vi "Connection Handler Worker.vi"(9 "Additional Data":variant, 10 "connection ID":T1, 11 "TCP Server Refnum":refnum<class "JKI TCP Server.lvclass">) -> ()   [LabVIEW 2020, in "CSM-TCP-Router.lvlib"]
uses:
  CSM-TCP-Router.lvlib
  <vilib>/addons/_JKI.lib/_JKI_lib_TCP_Server.llb/TCP Server Connection Session ID Cluster.ctl
  <vilib>/addons/_JKI.lib/_JKI_lib_TCP_Server.llb/JKI TCP Server.lvclass
  tcp-msg type.ctl
  20ff867f-262a-4864-b042-c50abd455195.vi
  9f8653f6-ccbf-4dca-88e7-a4c531b7661f.vi
  bd168d05-2ccd-4f69-90c9-be1b4e621865.vi
  316abe05-dd11-44a4-98b3-32ea1594dc48.vi
  a7f8194b-54d4-448d-8a65-d0b66a8fd47c.vi
  8a9da1d4-9237-4126-a3a1-8a9d876b672d.vi
  66683ee4-8938-4a2b-95b9-1d8ed72716c9.vi
  <userlib>/_NEVSTOP/Communicable State Machine(CSM)/AdvanceAPI/CSM - Revert Arguments-Safe String.vi
  <userlib>/_NEVSTOP/Communicable State Machine(CSM)/AdvanceAPI/CSM - Make String Arguments Safe.vi
  <userlib>/_NEVSTOP/Communicable State Machine(CSM)/AdvanceAPI/CSM - Compact Multiple States.vi
  <userlib>/_NEVSTOP/Communicable State Machine(CSM)/AdvanceAPI/CSM - Keywords.vi
  <userlib>/_NEVSTOP/Communicable State Machine(CSM)/addons/API-String-Arugments-Support/_Support/Data To API String Arguments.vi
  <userlib>/_NEVSTOP/Communicable State Machine(CSM)/_Shared/Trim Single-line Text.vi
  <userlib>/_NEVSTOP/Communicable State Machine(CSM)/addons/API-String-Arugments-Support/_Support/Query Data as API String Arguments(variant).vi
  <userlib>/_NEVSTOP/Communicable State Machine(CSM)/addons/API-String-Arugments-Support/_Support/Convert API String Arguments to Data(variant).vi
  <userlib>/_NEVSTOP/Communicable State Machine(CSM)/Communicable State Machine.lvlib
  <userlib>/_NEVSTOP/Communicable State Machine(CSM)/_csmHelper/API with lvcsm Support/CSM-Helper API with lvcsm Support.lvlib
  <userlib>/_NEVSTOP/Communicable State Machine(CSM)/_Shared/CSM Shared.lvlib
  <userlib>/_NEVSTOP/Communicable State Machine(CSM)/AdvanceAPI/CSM - Broadcast Message Type.ctl
panel:
  out "State History":string
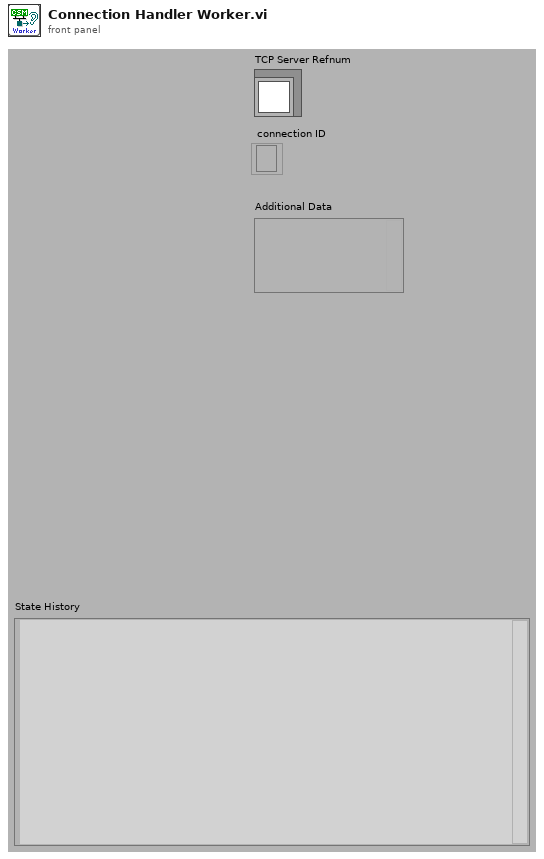
[diagram p1: front panel]
types:
  T1 = typedef "JKI TCP Server.lvclass/TCP Server Connection Session ID Cluster.ctl" = refnum<k5>
  T2 = typedef "CSM-TCP-Router.lvlib/tcp-msg type.ctl" = enum8{"info", "error", "cmd", "cmd-resp", "resp", "async-resp", "status", "interrupt"}
  T3 = typedef "Communicable State Machine.lvlib/CSM - Broadcast Message Type.ctl" = enum16{"<Null>", "Status", "Interrupt"}
  T4 = enum32{"Invalid", "Standard", "Closed", "Hidden", "Minimized", "Maximized"}
  T5 = enum32{"invalid app kind", "Development System", "Run Time System", "Student Edition", "Embedded LabVIEW", "Evaluation", "Custom"}
  T6 = typedef "Communicable State Machine.lvlib/_CSM_Response Source Message.ctl" = cluster{"‘State":string, "’Arguments":string, "’Error":errorcluster}
  T7 = cluster{"Current VI Reference":refnum<vi>, "Close Panel on Exit?":bool}
  T8 = cluster{"Core":cluster{"Current VI Reference":refnum<vi>, "Close Panel on Exit?":bool}, "Your Boolean data":bool}
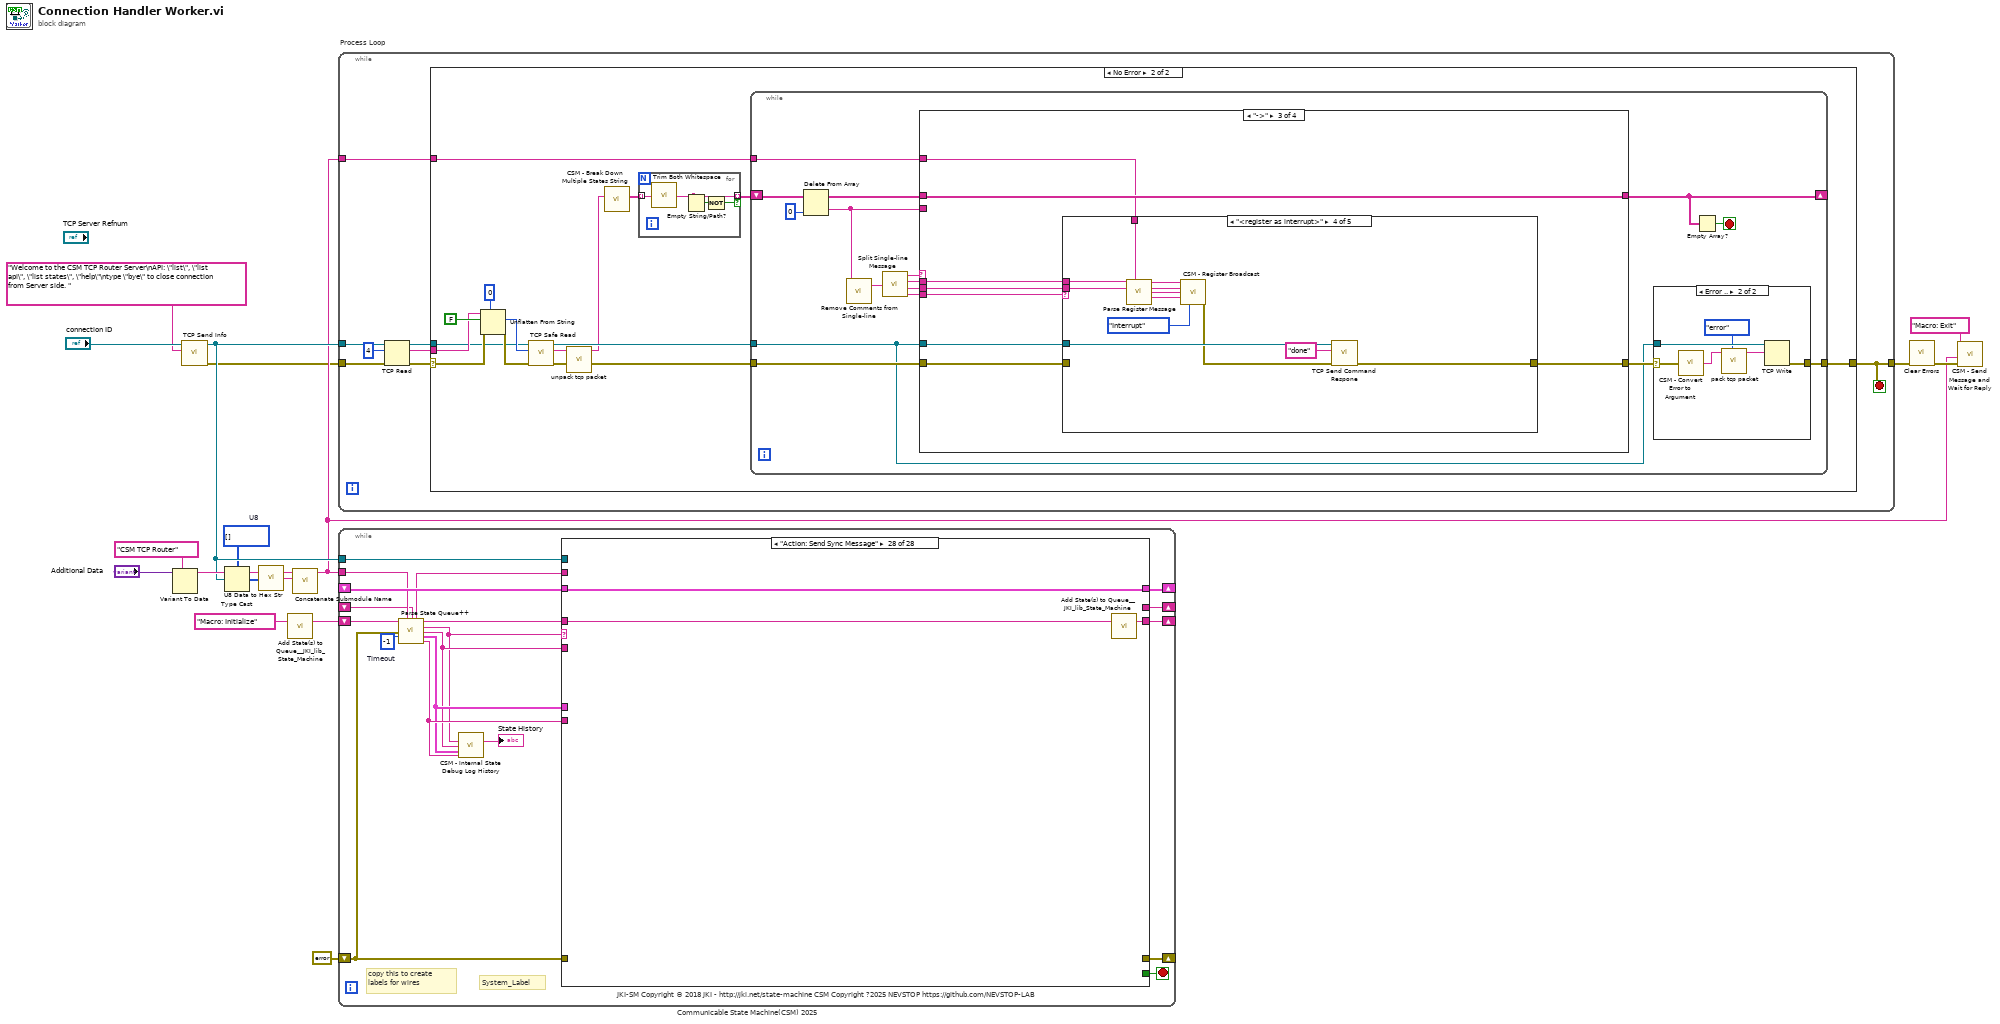
[diagram p0: block diagram]
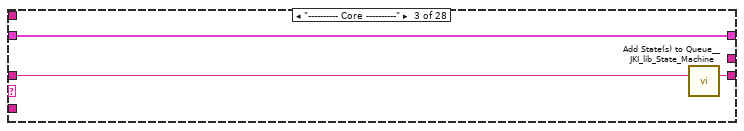
[diagram p4: hidden frame]
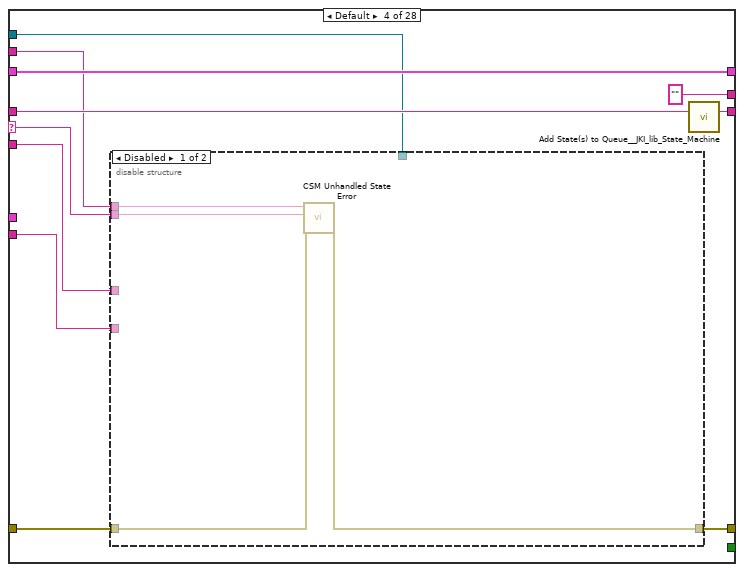
[diagram p5: hidden frame]
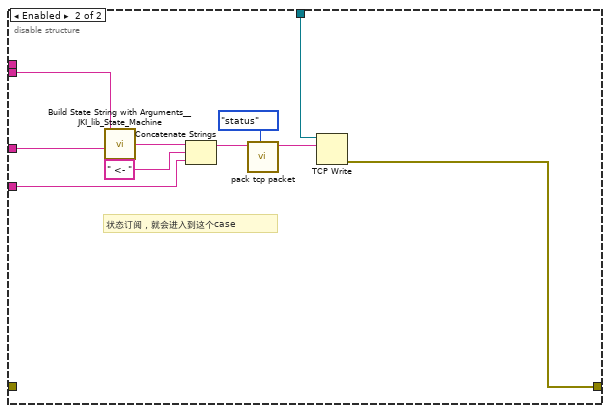
[diagram p6: hidden frame]
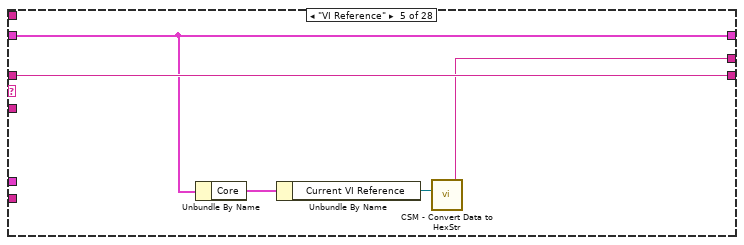
[diagram p7: hidden frame]
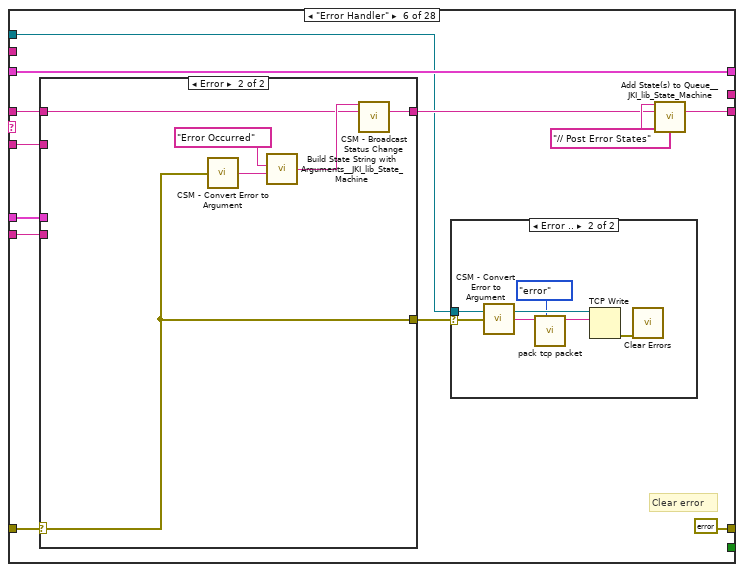
[diagram p8: hidden frame]
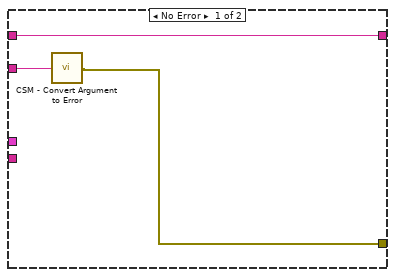
[diagram p10: hidden frame]
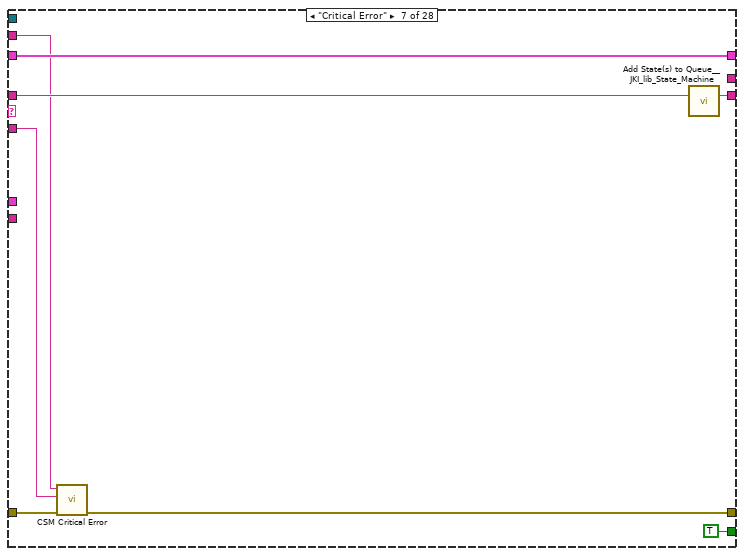
[diagram p11: hidden frame]
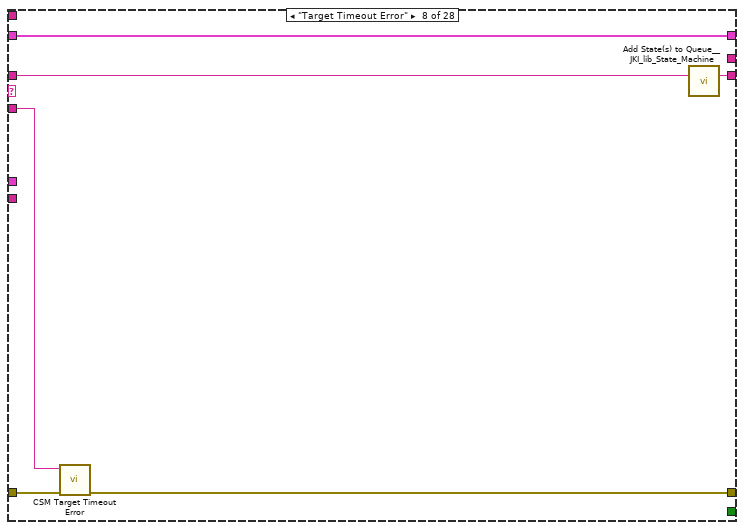
[diagram p12: hidden frame]
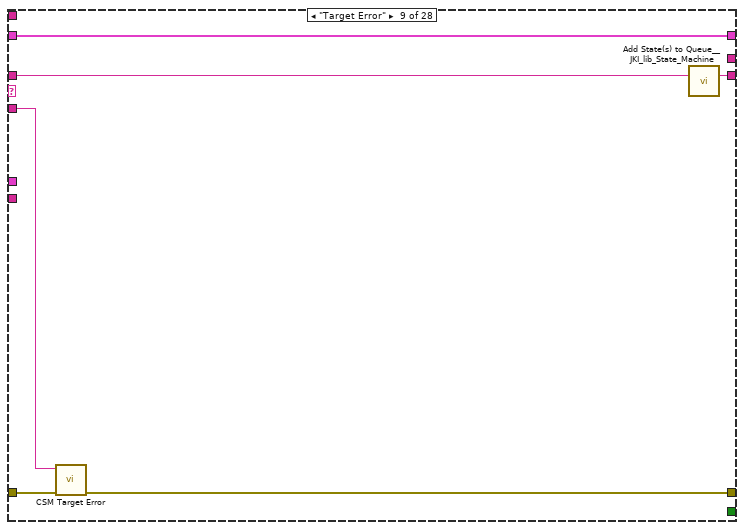
[diagram p13: hidden frame]
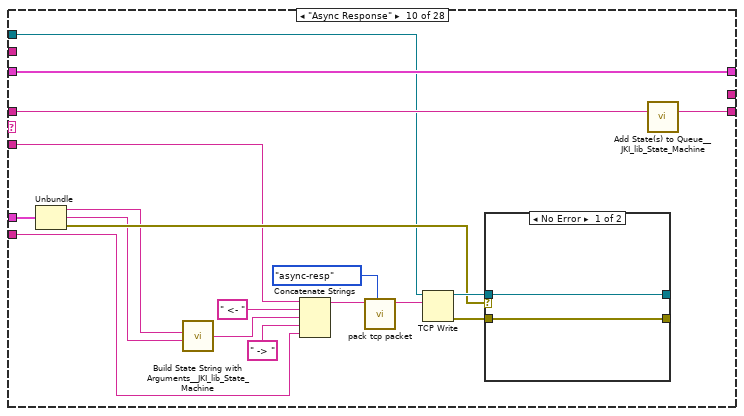
[diagram p14: hidden frame]
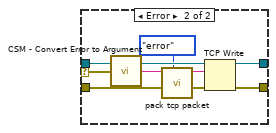
[diagram p15: hidden frame]
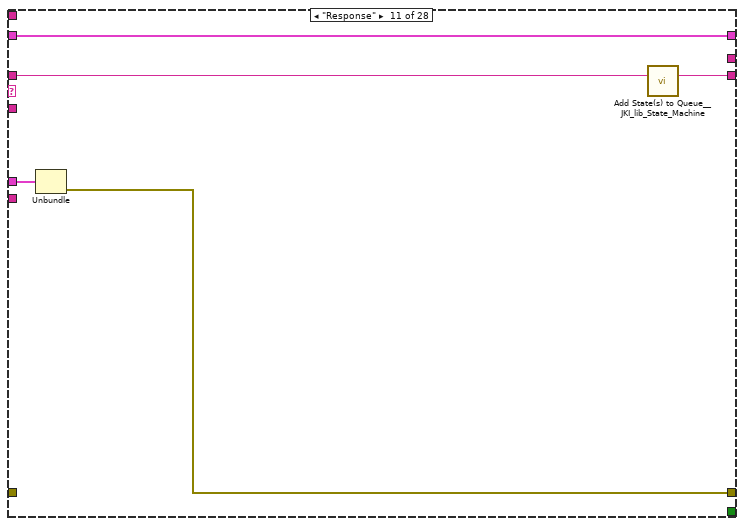
[diagram p16: hidden frame]
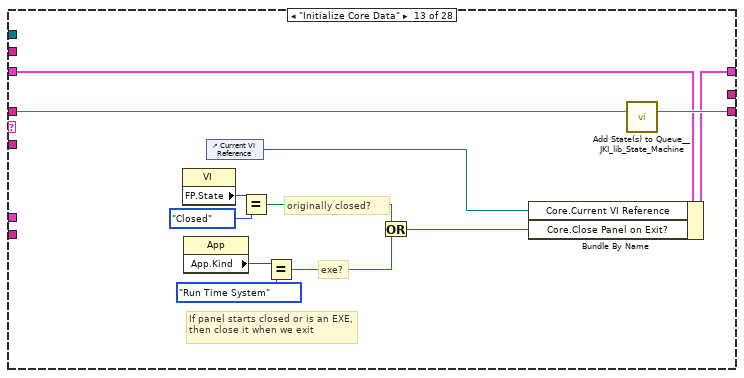
[diagram p18: hidden frame]
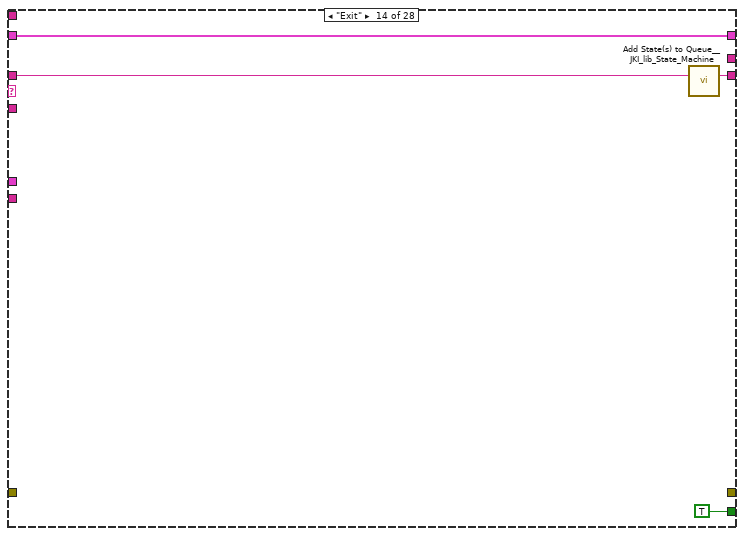
[diagram p19: hidden frame]
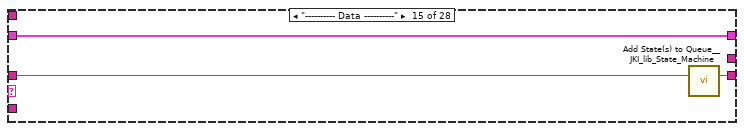
[diagram p20: hidden frame]
diagram:
  w5 = u8[] []  # U8
  n1 = Variant To Data(type="CSM TCP Router" ("Name(\"\" to use uuid)"), Variant="Additional Data") -> (data=w9:string)  [unwired: 1 in, 1 out]
  n2 = call "TCP Send Info.vi"("data in"="Welcome to the CSM TCP Router Server\nAPI: \"list\", \"list api\", \"list states\", \"help\"\ntype \"bye\" to close connection from Server side. ", "TCP Network Connection in"="connection ID") -> ("error out"=w2:errorcluster, "TCP Network Connection out"=w7:T1)  [unwired: 8 in]
  n3 = Type Cast(type=w5, x=w7) -> (*(type *) &x=w4:u8[])
  n4 = call <userlib>:"U8 Data to Hex Str.vi"("U8 Data[]"=w4) -> ("HEX String (0-9,A-F)"=w6:string)
  n5 = call <vilib>:"Add State(s) to Queue__JKI_lib_State_Machine.vi"("State(s) in (\"\")"="Macro: Initialize" ("Init States(\"Macro: Initialize\")")) -> ("States Out"=w15:string)  [unwired: 14 in]
  n6 = call <userlib>:"Concatenate Submodule Name.vi"("Module Name"=w6, "Group Name"=w9) -> ("Submodule Name"=w3:string)  [unwired: 9 in]
  n7 = while "Process Loop" {
    tunnel: w7 -> [w25]
    tunnel: [w21] -> w13
    tunnel: w3 -> [w20]
    tunnel: w2 -> [w18]
    stop <- w21 stop-if-true
    n8 = TCP Read(connection ID=w25, bytes to read=4, error in (no error)=w18) -> (connection ID out=w24:T1, data out=w22:string, error out=w23:errorcluster)  [unwired: 2 in]
    n9 = case shown="No Error" w23 {
      selector: w23 -> [w27 w37]
      tunnel: w24 -> [_ w30]
      tunnel: w22 -> [_ w38]
      tunnel: [w26 w44] -> w21
      tunnel: w20 -> [_ w41]
      frame Error {
        n10 = Unbundle By Name(w27) -> ("code"=w28:i32)
        n11 = case shown="56" w28 {
          tunnel: w27 -> [w29 _]
          tunnel: [w29 _] -> w26
          frame 0, Default {
          }
          frame 56 {
          }
        }
      }
      frame No Error {
        n12 = Unflatten From String(type=0, binary string=w38, data includes array or string size? (T)=FALSE, error in (no error)=w37) -> (value=w33:i32, error out=w36:errorcluster)  [unwired: 2 out]
        n13 = call "TCP Safe Read.vi"("error in (no error)"=w36, "bytes to read"=w33, "TCP Network Connection in"=w30) -> ("error out"=w35:errorcluster, "String"=w32:string, "TCP Network Connection out"=w34:refnum<k5>)  [unwired: 6 in]
        n14 = call "unpack tcp packet.vi"("TCP Pack"=w32) -> ("String"=w31:string)  [unwired: 9 in, 1 out]
        n15 = call <userlib>:"CSM - Break Down Multiple States String.vi"("States"=w31) -> ("Multiple States"=w43:string[])  [unwired: 10 in]
        n16 = for {
          tunnel: w43 -> [w48] mode=indexing
          tunnel: [w47] -> w42 mode=indexing if=w45
          n17 = call <userlib>:"Trim Both Whitespace.vi"("String"=w48) -> ("Trimmed String"=w47:string)  [unwired: 1 in]
          n18 = Empty String/Path?(string/path=w47) -> (empty?=w46:bool)
          n19 = Not(x=w46) -> (.not. x?=w45:bool)
        }
        n20 = while {
          tunnel: w34 -> [w51]
          tunnel: w35 -> [w64]
          tunnel: [w52] -> w44
          shift-right: [w54] -> _
          shift-left: w42 -> [w58]
          tunnel: w41 -> [w49]
          stop <- w55 stop-if-true
          n21 = Delete From Array(array=w58, index=0) -> (deleted portion=w50:string, array with subset deleted=w57:string[])  [unwired: 1 in]
          n22 = call <userlib>:"Remove Comments from Single-line.vi"("single-line text"=w50) -> ("single-line text without comments"=w63:string)  [unwired: 2 in]
          n23 = call <userlib>:"Split Single-line Message.vi"("single-line text"=w63) -> ("operator"=w62:string, "state"=w61:string, "args"=w60:string, "source/target"=w59:string)  [unwired: 6 in]
          n24 = case shown="\"->\"" w62 {
            selector: w62 -> [w75 _ _ _]
            tunnel: w51 -> [w81 w192 w196 w263]
            tunnel: [w80 w191 w200 w267] -> w53
            tunnel: w64 -> [w79 w184 w198 w265]
            tunnel: w61 -> [w78 w186 w195 w262]
            tunnel: w60 -> [w77 w185 w194 w261]
            tunnel: w59 -> [w76 w187 w193 w260]
            tunnel: [w74 w189 w199 w266] -> w54
            tunnel: w57 -> [w73 w189 w199 w266]
            tunnel: w50 -> [_ _ _ _]
            tunnel: w49 -> [w72 w188 w197 w264]
            frame Default {
              n25 = case shown="Default" w78 {
                selector: w78 -> [w89 _ _ _ _ _ _ _]
                tunnel: w81 -> [w92 w97 w107 w120 w133 w146 w160 w180]
                tunnel: [w91 errorcluster {"status"=TRUE, "code"=0, "source"=""} ("error out") w102 w119 w132 w145 w162 w181] -> w80
                tunnel: w79 -> [w84 w98 w106 _ _ _ w161 w178]
                tunnel: w77 -> [w90 _ _ w115 w128 w141 _ _]
                tunnel: w76 -> [_ _ _ _ _ _ _ _]
                tunnel: w75 -> [_ _ _ _ _ _ _ _]
                tunnel: [w88 w95 w101 w118 w131 w144 w168 w182] -> w74
                tunnel: w73 -> [w88 w95 w101 w118 w131 w144 w168 w182]
                tunnel: w72 -> [_ _ _ w114 w127 w140 w163 _]
                frame Default {
                  n26 = call <vilib>:"Build State String with Arguments__JKI_lib_State_Machine.vi"("Arguments (\"\")"=w90, "State"=w89) -> ("State with Arguments"=w85:string)  [unwired: 4 in]
                  n27 = Format Into String(format string="You typed \"%s\", which is not recognized as a command", w85) -> (resulting string=w86:string)  [unwired: 2 in, 1 out]
                  n28 = call "pack tcp packet.vi"("tcp-message-type"=tcp-msg_type."error", "String"=w86) -> ("TCP Pack"=w83:string)  [unwired: 9 in]
                  n29 = TCP Write(connection ID=w92, data in=w83, error in (no error)=w84) -> (error out=w91:errorcluster)  [unwired: 1 in, 2 out]
                }
                frame "bye", "exit", "quit" {
                  n30 = call "TCP Send Info.vi"("error in (no error)"=w98, "data in"="Good bye.\r\n", "TCP Network Connection in"=w97) -> ("error out"=w94:errorcluster, "TCP Network Connection out"=w93:T1)  [unwired: 7 in]
                  n31 = TCP Close Connection(connection ID=w93, error in (no error)=w94) -> ()  [unwired: 1 in, 2 out]
                }
                frame "list", "list CSM", "List CSMs" {
                  n32 = call <userlib>:"CSM - List Modules.vi"("Error In"=w106) -> ("error out"=w104:errorcluster, "Module Names"=w105:string[])  [unwired: 9 in]
                  n33 = call "Convert Data To API String Arguments.vim"("error in (no error)"=w104, "Data"=w105) -> ("error out"=w103:errorcluster, "API String"=w100:string)  [unwired: 6 in]
                  n34 = call "TCP Send Response.vi"("error in (no error)"=w103, "Response"=w100, "connection ID"=w107) -> ("error out"=w102:errorcluster)  [unwired: 7 in, 1 out]
                }
                frame "list API", "list interface" {
                  n35 = call <userlib>:"CSM - Check If Module Exists.vi"("CSM Name"=w115) -> ("error out"=w117:errorcluster, "Exist?"=w112:bool, "CSM Name (Dup)"=w116:string)  [unwired: 8 in]
                  n36 = call "Error If Module Not Exist.vi"("Error in"=w117, "Module Exist?"=w112) -> ("Error out"=w113:errorcluster)  [unwired: 9 in]
                  n37 = call <userlib>:"Read CSM API with lvcsm Support.vi"("Current Module (\"\" to Generate an ID)"=w114, "error in (no error)"=w113, "CSM Name"=w116) -> ("error out"=w110:errorcluster, "CSMAPI List"=w109:string[])  [unwired: 7 in]
                  n38 = call "Convert Data To API String Arguments.vim"("error in (no error)"=w110, "Data"=w109) -> ("error out"=w111:errorcluster, "API String"=w108:string)  [unwired: 6 in]
                  n39 = call "TCP Send Response.vi"("error in (no error)"=w111, "Response"=w108, "connection ID"=w120) -> ("error out"=w119:errorcluster)  [unwired: 7 in, 1 out]
                }
                frame "List State", "List States" {
                  n40 = call <userlib>:"CSM - Check If Module Exists.vi"("CSM Name"=w128) -> ("error out"=w130:errorcluster, "Exist?"=w125:bool, "CSM Name (Dup)"=w129:string)  [unwired: 8 in]
                  n41 = call "Error If Module Not Exist.vi"("Error in"=w130, "Module Exist?"=w125) -> ("Error out"=w126:errorcluster)  [unwired: 9 in]
                  n42 = call <userlib>:"Read CSM States with lvcsm Support.vi"("Current Module (\"\" to Generate an ID)"=w127, "error in (no error)"=w126, "CSM Name"=w129) -> ("error out"=w121:errorcluster, "CSMAPI List"=w122:string[])  [unwired: 7 in]
                  n43 = call "Convert Data To API String Arguments.vim"("error in (no error)"=w121, "Data"=w122) -> ("error out"=w124:errorcluster, "API String"=w123:string)  [unwired: 6 in]
                  n44 = call "TCP Send Response.vi"("error in (no error)"=w124, "Response"=w123, "connection ID"=w133) -> ("error out"=w132:errorcluster)  [unwired: 7 in, 1 out]
                }
                frame "help" {
                  n45 = call <userlib>:"CSM - Check If Module Exists.vi"("CSM Name"=w141) -> ("error out"=w143:errorcluster, "Exist?"=w138:bool, "CSM Name (Dup)"=w142:string)  [unwired: 8 in]
                  n46 = call "Error If Module Not Exist.vi"("Error in"=w143, "Module Exist?"=w138) -> ("Error out"=w139:errorcluster)  [unwired: 9 in]
                  n47 = disable-structure shown="Enabled" {
                    disable-tunnel: w139 -> [w153 w158]
                    disable-tunnel: w142 -> [w152 w157]
                    disable-tunnel: [w150 w155] -> w135
                    disable-tunnel: [w148 w154] -> w134
                    disable-tunnel: w140 -> [w147 w156]
                    frame Disabled {
                      n48 = call <userlib>:"CSM - Module VI Reference.vi"("Current Module (\"\" to Generate an ID)"=w147, "error in (no error)"=w153, "CSM Name"=w152) -> ("error out"=w151:errorcluster, "CSM Module VIRef"=w149:refnum<vi>)  [unwired: 7 in]
                      n49 = property class="VI"(reference=w149, error in=w151) -> (error out=w150:errorcluster, "Description"=w148:string)  [unwired: 1 out]
                    }
                    frame Enabled {
                      n50 = call "Read CSM Doc.vi"("Current Module(\"\" to generate a ID)"=w156, "error in (no error)"=w158, "CSM Name"=w157) -> ("Error out"=w155:errorcluster, "CSM Doc"=w154:string)  [unwired: 7 in]
                    }
                  }
                  n51 = call "Convert Data To API String Arguments.vim"("error in (no error)"=w135, "Data"=w134) -> ("error out"=w137:errorcluster, "API String"=w136:string)  [unwired: 6 in]
                  n52 = call "TCP Send Response.vi"("error in (no error)"=w137, "Response"=w136, "connection ID"=w146) -> ("error out"=w145:errorcluster)  [unwired: 7 in, 1 out]
                }
                frame "Refresh lvcsm" {
                  n53 = call <userlib>:"CSM - List Modules.vi"("Error In"=w161) -> ("error out"=w167:errorcluster, "Module Names"=w166:string[])  [unwired: 9 in]
                  n54 = for {
                    tunnel: w167 -> [w177]
                    tunnel: w166 -> [w170] mode=indexing
                    tunnel: [w172] -> w165 mode=indexing
                    tunnel: w163 -> [w171]
                    n55 = call <userlib>:"Read CSM States with lvcsm Support.vi"("Current Module (\"\" to Generate an ID)"=w171, "error in (no error)"=w177, "Force? (F)"=TRUE ("Force?(F)"), "CSM Name"=w170) -> ("error out"=w176:errorcluster)  [unwired: 6 in, 1 out]
                    n56 = call <userlib>:"Read CSM API with lvcsm Support.vi"("Current Module (\"\" to Generate an ID)"=w171, "error in (no error)"=w176, "Force? (F)"=TRUE ("Force?(F)"), "CSM Name"=w170) -> ("error out"=w173:errorcluster)  [unwired: 6 in, 1 out]
                    n57 = call "Read CSM Doc.vi"("Current Module(\"\" to generate a ID)"=w171, "error in (no error)"=w173, "Force?(F)"=TRUE, "CSM Name"=w170) -> ("Error out"=w172:errorcluster)  [unwired: 6 in, 1 out]
                  }
                  n58 = Merge Errors(w165) -> (w164:errorcluster)
                  n59 = call "TCP Send Response.vi"("error in (no error)"=w164, "Response"="", "connection ID"=w160) -> ("error out"=w162:errorcluster)  [unwired: 7 in, 1 out]
                }
                frame "ping" {
                  n60 = call "TCP Send Response.vi"("error in (no error)"=w178, "Response"="pong", "connection ID"=w180) -> ("error out"=w181:errorcluster)  [unwired: 7 in, 1 out]
                }
              }
            }
            frame "-@" {
              n61 = call <userlib>:"CSM - Send Message and Wait for Reply.vi"("Current Module (\"\" to Generate an ID)"=w188, "Error In (No Error)"=w184, "Target Module"=w187, "Arguments (\"\")"=w185, "State"=w186) -> ("error out"=w183:errorcluster, "Response"=w190:string)  [unwired: 4 in, 1 out]
              n62 = call "TCP Send Response.vi"("error in (no error)"=w183, "Response"=w190, "connection ID"=w192) -> ("error out"=w191:errorcluster)  [unwired: 7 in, 1 out]
            }
            frame "->" {
              n63 = case shown="\"<register as interrupt>\"" w193 {
                selector: w193 -> [_ _ _ _ w250]
                tunnel: [w201 w213 w225 w237 w256] -> w200
                tunnel: w198 -> [_ _ _ _ w255]
                tunnel: w197 -> [w209 w220 w232 w244 w254]
                tunnel: w196 -> [w203 w215 w227 w239 w253]
                tunnel: w195 -> [w210 w221 w233 w245 w252]
                tunnel: w194 -> [w211 w222 w234 w246 w251]
                frame "<unregister>" {
                  n64 = call <userlib>:"Parse Unregister Message.vi"("State"=w210, "Module Name"=w209, "Args"=w211) -> ("Target"=w207:string, "Source"=w208:string, "Status"=w206:string, "Api"=w205:string)  [unwired: 8 in, 1 out]
                  n65 = call <userlib>:"CSM - Unregister Broadcast.vi"("CSM Name(Empty for Broadcast Event)"=w207, "Source CSM Name (* as Default)"=w208, "Trigger"=w206, "API (\"*\" as Default)"=w205) -> ("error out"=w202:errorcluster)  [unwired: 10 in, 1 out]
                  n66 = call "TCP Send Command Respone.vi"("error in (no error)"=w202, "Response"="done", "connection ID"=w203) -> ("error out"=w201:errorcluster)  [unwired: 7 in, 1 out]
                }
                frame "<register>" {
                  n67 = call <userlib>:"Parse Register Message.vi"("State"=w221, "Module Name"=w220, "Args"=w222) -> ("Target"=w218:string, "Source"=w219:string, "Status"=w217:string, "Api"=w216:string)  [unwired: 8 in, 1 out]
                  n68 = call <userlib>:"CSM - Register Broadcast.vi"("CSM Name(Empty for Broadcast Event)"=w218, "Source CSM Name (* as Default)"=w219, "Trigger"=w217, "API (If \"\", Same as Trigger)"=w216) -> ("error out"=w214:errorcluster)  [unwired: 10 in, 1 out]
                  n69 = call "TCP Send Command Respone.vi"("error in (no error)"=w214, "Response"="done", "connection ID"=w215) -> ("error out"=w213:errorcluster)  [unwired: 7 in, 1 out]
                }
                frame "<register as status>" {
                  n70 = call <userlib>:"Parse Register Message.vi"("State"=w233, "Module Name"=w232, "Args"=w234) -> ("Target"=w230:string, "Source"=w231:string, "Status"=w229:string, "Api"=w228:string)  [unwired: 8 in, 1 out]
                  n71 = call <userlib>:"CSM - Register Broadcast.vi"("CSM Name(Empty for Broadcast Event)"=w230, "Source CSM Name (* as Default)"=w231, "Trigger"=w229, "API (If \"\", Same as Trigger)"=w228, "Priority (No Change)"=CSM_-_Broadcast_Message_Type."Status") -> ("error out"=w226:errorcluster)  [unwired: 9 in, 1 out]
                  n72 = call "TCP Send Command Respone.vi"("error in (no error)"=w226, "Response"="done", "connection ID"=w227) -> ("error out"=w225:errorcluster)  [unwired: 7 in, 1 out]
                }
                frame "<register as interrupt>" {
                  n73 = call <userlib>:"Parse Register Message.vi"("State"=w245, "Module Name"=w244, "Args"=w246) -> ("Target"=w242:string, "Source"=w243:string, "Status"=w241:string, "Api"=w240:string)  [unwired: 8 in, 1 out]
                  n74 = call <userlib>:"CSM - Register Broadcast.vi"("CSM Name(Empty for Broadcast Event)"=w242, "Source CSM Name (* as Default)"=w243, "Trigger"=w241, "API (If \"\", Same as Trigger)"=w240, "Priority (No Change)"=CSM_-_Broadcast_Message_Type."Interrupt") -> ("error out"=w238:errorcluster)  [unwired: 9 in, 1 out]
                  n75 = call "TCP Send Command Respone.vi"("error in (no error)"=w238, "Response"="done", "connection ID"=w239) -> ("error out"=w237:errorcluster)  [unwired: 7 in, 1 out]
                }
                frame Default {
                  n76 = call <userlib>:"CSM - Request CSM to Post Message.vi"("Module Name"=w254, "Target Module (\"\" By Default)"=w250, "Arguments (\"\")"=w251, "State"=w252) -> ("error out"=w247:errorcluster)  [unwired: 7 in]
                  n77 = Merge Errors(w255, w247) -> (w248:errorcluster)
                  n78 = call "TCP Send Command Respone.vi"("error in (no error)"=w248, "Response"="Message posted", "connection ID"=w253) -> ("error out"=w256:errorcluster)  [unwired: 7 in, 1 out]
                }
              }
            }
            frame "->|" {
              n79 = call <userlib>:"CSM - Post Message.vi"("Current Module (\"\" to Generate an ID)"=w264, "Target Module"=w260, "Arguments (\"\")"=w261, "State"=w262) -> ("error out"=w258:errorcluster)  [unwired: 7 in]
              n80 = call "Synchronize Data Flow.vim"("input 2"=w265, "input 1"=w258) -> ("output 2"=w259:errorcluster)  [unwired: 2 in, 3 out]
              n81 = call "TCP Send Command Respone.vi"("error in (no error)"=w259, "Response"="No-Rep Message Posted", "connection ID"=w263) -> ("error out"=w267:errorcluster)  [unwired: 7 in, 1 out]
            }
          }
          n82 = case shown="Error .." w53 {
            selector: w53 -> [w65 w68]
            tunnel: w51 -> [_ w71]
            tunnel: [w65 w70] -> w52
            frame No Error {
            }
            frame Error {
              n83 = call <userlib>:"CSM - Convert Error to Argument.vi"("Error"=w68) -> ("Argument"=w69:string)  [unwired: 4 in]
              n84 = call "pack tcp packet.vi"("tcp-message-type"=tcp-msg_type."error", "String"=w69) -> ("TCP Pack"=w67:string)  [unwired: 9 in]
              n85 = TCP Write(connection ID=w71, data in=w67) -> (error out=w70:errorcluster)  [unwired: 2 in, 2 out]
            }
          }
          n86 = Empty Array?(array=w54) -> (empty?=w55:bool)
        }
      }
    }
  }
  n87 = while "Communicable State Machine(CSM) 2025" {
    shift-right: [w281] -> _
    shift-left: _ -> [w280]
    shift-right: [w284] -> _
    shift-left: errorcluster {"status"=FALSE, "code"=0, "source"=""} ("error out") -> [w270]
    shift-right: [w283] -> _
    shift-left: w15 -> [w285]
    tunnel: w3 -> [w277]
    shift-right: [w278] -> _
    shift-left: _ -> [w272]
    tunnel: w7 -> [w268]
    stop <- w282 stop-if-true
    w279 = -1  # Timeout
    # "copy this to create labels for wires"
    # "System_Label"
    # "JKI-SM Copyright © 2018 JKI - http://jki.net/state-machine CSM Copyright ?2025 NEVSTOP https://github.com/NEVSTOP-LAB"
    n88 = call <userlib>:"Parse State Queue++.vi"("State Queue"=w285, "Name (\"\" to Use UUID)"=w277, "Response Arguments"=w272, "Previous Error"=w270, "Dequeue (1 ms)"=w279) -> ("Name Used"=w271:string, "Remaining States"=w286:string, "Current State"=w273:string, "Arguments"=w274:string, "Additional Information"=w275:T6, "Source CSM"=w276:string)  [unwired: 5 in]
    n89 = call <userlib>:"CSM - Internal State Debug Log History.vi"("State"=w273, "Arguments (\"\")"=w274, ">> Response Source Message >>"=w275, "Source (\"\")"=w276) -> ("Debug Log"=→"State History":string)  [unwired: 11 in]
    n90 = case shown="\"Action: Send Sync Message\"" w273 {
      selector: w273 -> [_ _ _ w299 _ _ _ _ _ _ _ _ _ _ _ _ _ _ _ _ _ _ _ _ _ _ _ _]
      tunnel: w286 -> [w287 w290 w293 w302 w323 w329 w357 w363 w369 w386 w401 w405 w417 w421 w424 w429 w435 w440 w442 w447 w450 w454 w458 w460 w463 w467 w472 w475]
      tunnel: w274 -> [_ _ _ w295 _ w328 w351 w360 w366 w378 _ _ _ _ _ _ w430 w439 _ _ _ _ _ _ _ w465 _ _]
      tunnel: w280 -> [w288 w289 w291 w300 w320 w334 w355 w361 w367 w387 w402 w404 w411 w419 w422 _ w434 w438 w441 w443 w448 w452 w456 w459 w462 w466 w470 w473]
      tunnel: [_ _ _ w304 _ errorcluster {"status"=FALSE, "code"=0, "source"=""} ("error out") w358 w359 w365 _ w399 _ _ _ _ _ w431 w436 _ w444 _ _ _ _ _ _ _ _] -> w284
      tunnel: w270 -> [_ _ _ w303 _ w332 w353 w364 w370 _ _ _ _ _ _ _ _ _ _ _ _ _ _ _ _ _ _ _]
      tunnel: [w287 w290 w292 w301 w323 w330 w356 w362 w368 w388 w403 w405 w416 w420 w423 w428 w435 w440 w442 w446 w449 w453 w457 w460 w463 w467 w471 w474] -> w283
      tunnel: [_ _ _ _ _ _ TRUE _ _ _ _ _ _ TRUE _ _ _ _ _ _ _ _ _ _ _ _ _ _] -> w282
      tunnel: [w288 w289 w291 w300 w320 w334 w355 w361 w367 w387 w402 w404 w415 w419 w422 w427 w433 w437 w441 w443 w448 w452 w456 w459 w462 w466 w470 w473] -> w281
      tunnel: w276 -> [_ _ _ w294 _ w327 _ _ _ w371 _ _ _ _ _ _ _ _ _ _ _ _ _ _ _ _ _ _]
      tunnel: w275 -> [_ _ _ _ _ w326 _ _ _ w385 w400 _ _ _ _ _ _ _ _ _ _ _ _ _ _ _ _ _]
      tunnel: [_ _ _ "" w319 _ _ _ _ _ _ _ _ _ _ _ w432 _ _ _ _ _ _ _ "API1 Response" w464 _ _] -> w278
      tunnel: w271 -> [_ _ _ w297 _ _ w352 _ _ _ _ _ _ _ _ _ _ _ _ _ _ _ _ _ _ _ _ _]
      tunnel: w268 -> [_ _ _ w296 _ w324 _ _ _ w379 _ _ _ _ _ _ _ _ _ _ _ _ _ _ _ _ _ _]
      frame "", "Idle" {
      }
      frame "CSM Documentation" {
      }
      frame "---------- Core ----------" {
        n91 = call <vilib>:"Add State(s) to Queue__JKI_lib_State_Machine.vi"("State(s) in (\"\")"=w293) -> ("States Out"=w292:string)  [unwired: 14 in]
      }
      frame Default {
        n92 = disable-structure shown="Disabled" {
          disable-tunnel: [w308 w309] -> w304
          disable-tunnel: w303 -> [w307 _]
          disable-tunnel: w299 -> [w306 w313]
          disable-tunnel: w297 -> [w305 _]
          disable-tunnel: w296 -> [_ w314]
          disable-tunnel: w295 -> [_ w312]
          disable-tunnel: w294 -> [_ w310]
          frame Disabled {
            n93 = call <userlib>:"CSM Unhandled State Error.vi"("error in (no error)"=w307, "Undefined State"=w306, "CSM Name"=w305) -> ("error out"=w308:errorcluster)  [unwired: 8 in]
          }
          frame Enabled {
            # "状态订阅，就会进入到这个case"
            n94 = call <vilib>:"Build State String with Arguments__JKI_lib_State_Machine.vi"("Arguments (\"\")"=w312, "State"=w313) -> ("State with Arguments"=w311:string)  [unwired: 4 in]
            n95 = Concatenate Strings(w311, " <- " ("string"), w310) -> (w316:string)
            n96 = call "pack tcp packet.vi"("tcp-message-type"=tcp-msg_type."status", "String"=w316) -> ("TCP Pack"=w318:string)  [unwired: 9 in]
            n97 = TCP Write(connection ID=w314, data in=w318) -> (error out=w309:errorcluster)  [unwired: 2 in, 2 out]
          }
        }
        n98 = call <vilib>:"Add State(s) to Queue__JKI_lib_State_Machine.vi"("State(s) in (\"\")"=w302) -> ("States Out"=w301:string)  [unwired: 14 in]
      }
      frame "VI Reference" {
        n99 = Unbundle By Name(w320) -> ("Core"=w322:T7)
        n100 = Unbundle By Name(w322) -> ("Current VI Reference"=w321:refnum<vi>)
        n101 = call <userlib>:"CSM - Convert Data to HexStr.vi"("Variant"=w321) -> ("HEX String (0-9,A-F)"=w319:string)  [unwired: 8 in]
      }
      frame "Error Handler" {
        # "Clear error"
        n102 = case shown="Error" w332 {
          selector: w332 -> [_ w345]
          tunnel: [w344 w347] -> w331
          tunnel: w329 -> [w344 w346]
          tunnel: w328 -> [w343 _]
          tunnel: w327 -> [_ _]
          tunnel: w326 -> [_ _]
          tunnel: [w342 w345] -> w325
          frame No Error {
            n103 = call <userlib>:"CSM - Convert Argument to Error.vi"("Argument"=w343) -> ("Error"=w342:errorcluster)  [unwired: 4 in]
          }
          frame Error {
            n104 = call <userlib>:"CSM - Convert Error to Argument.vi"("Error"=w345) -> ("Argument"=w349:string)  [unwired: 4 in]
            n105 = call <vilib>:"Build State String with Arguments__JKI_lib_State_Machine.vi"("Arguments (\"\")"=w349, "State"="Error Occurred" ("Status with Arguments")) -> ("State with Arguments"=w348:string)  [unwired: 4 in]
            n106 = call <userlib>:"CSM - Broadcast Status Change.vi"("Status With Arguments"=w348, "State Queue"=w346) -> ("Remaining States"=w347:string)  [unwired: 13 in]
          }
        }
        n107 = case shown="Error .." w325 {
          selector: w325 -> [_ w339]
          tunnel: w324 -> [_ w341]
          frame No Error {
          }
          frame Error {
            n108 = call <userlib>:"CSM - Convert Error to Argument.vi"("Error"=w339) -> ("Argument"=w338:string)  [unwired: 4 in]
            n109 = call "pack tcp packet.vi"("tcp-message-type"=tcp-msg_type."error", "String"=w338) -> ("TCP Pack"=w337:string)  [unwired: 9 in]
            n110 = TCP Write(connection ID=w341, data in=w337) -> (error out=w340:errorcluster)  [unwired: 2 in, 2 out]
            n111 = call <vilib>:"Clear Errors.vi"("error in (no error)"=w340) -> ()  [unwired: 5 in, 2 out]
          }
        }
        n112 = call <vilib>:"Add State(s) to Queue__JKI_lib_State_Machine.vi"("State(s) in Front (\"\")"="// Post Error States", "State(s) in (\"\")"=w331) -> ("States Out"=w330:string)  [unwired: 13 in]
      }
      frame "Critical Error" {
        n113 = call <userlib>:"CSM Critical Error.vi"("error in (no error)"=w353, "Arugments (As Reason)"=w351, "CSM Name"=w352) -> ("error out"=w358:errorcluster)  [unwired: 8 in]
        n114 = call <vilib>:"Add State(s) to Queue__JKI_lib_State_Machine.vi"("State(s) in (\"\")"=w357) -> ("States Out"=w356:string)  [unwired: 14 in]
      }
      frame "Target Timeout Error" {
        n115 = call <userlib>:"CSM Target Timeout Error.vi"("error in (no error)"=w364, "Arguments (As CSM Name)"=w360) -> ("error out"=w359:errorcluster)  [unwired: 9 in]
        n116 = call <vilib>:"Add State(s) to Queue__JKI_lib_State_Machine.vi"("State(s) in (\"\")"=w363) -> ("States Out"=w362:string)  [unwired: 14 in]
      }
      frame "Target Error" {
        n117 = call <userlib>:"CSM Target Error.vi"("error in (no error)"=w370, "Arguments (As CSM Name)"=w366) -> ("error out"=w365:errorcluster)  [unwired: 9 in]
        n118 = call <vilib>:"Add State(s) to Queue__JKI_lib_State_Machine.vi"("State(s) in (\"\")"=w369) -> ("States Out"=w368:string)  [unwired: 14 in]
      }
      frame "Async Response" {
        n119 = Unbundle(w385) -> ("‘State"=w375:string, "’Arguments"=w374:string, "’Error"=w380:errorcluster)
        n120 = call <vilib>:"Build State String with Arguments__JKI_lib_State_Machine.vi"("Arguments (\"\")"=w374, "State"=w375) -> ("State with Arguments"=w373:string)  [unwired: 4 in]
        n121 = Concatenate Strings(w378, " <- " ("string"), w373, " -> " ("string"), w371) -> (w377:string)
        n122 = call "pack tcp packet.vi"("tcp-message-type"=tcp-msg_type."async-resp", "String"=w377) -> ("TCP Pack"=w384:string)  [unwired: 9 in]
        n123 = TCP Write(connection ID=w379, data in=w384) -> (connection ID out=w383:T1, error out=w382:errorcluster)  [unwired: 2 in, 1 out]
        n124 = case shown="No Error" w380 {
          selector: w380 -> [_ w395]
          tunnel: w382 -> [w390 w398]
          tunnel: w383 -> [w389 w397]
          tunnel: [w390 w396] -> _
          tunnel: [w389 w393] -> _
          frame No Error {
          }
          frame Error {
            n125 = call <userlib>:"CSM - Convert Error to Argument.vi"("Error"=w395) -> ("Argument"=w394:string)  [unwired: 4 in]
            n126 = call "pack tcp packet.vi"("tcp-message-type"=tcp-msg_type."error", "String"=w394) -> ("TCP Pack"=w392:string)  [unwired: 9 in]
            n127 = TCP Write(connection ID=w397, data in=w392, error in (no error)=w398) -> (connection ID out=w393:T1, error out=w396:errorcluster)  [unwired: 1 in, 1 out]
          }
        }
        n128 = call <vilib>:"Add State(s) to Queue__JKI_lib_State_Machine.vi"("State(s) in (\"\")"=w386) -> ("States Out"=w388:string)  [unwired: 14 in]
      }
      frame "Response" {
        n129 = Unbundle(w400) -> ("’Error"=w399:errorcluster)  [unwired: 2 out]
        n130 = call <vilib>:"Add State(s) to Queue__JKI_lib_State_Machine.vi"("State(s) in (\"\")"=w401) -> ("States Out"=w403:string)  [unwired: 14 in]
      }
      frame "Async Message Posted" {
      }
      frame "Initialize Core Data" {
        # "originally closed?"
        # "exe?"
        # "If panel starts closed or is an EXE, then close it when we exit"
        n131 = property class="VI"() -> ("FP.State"=w408:T4)  [unwired: 2 in, 2 out]
        n132 = property class="App"() -> ("App.Kind"=w414:T5)  [unwired: 2 in, 2 out]
        n133 = control-ref of="Current VI Reference"() -> (w409:refnum<vi>)
        n134 = Equal?(x=w408, y=T4."Closed" ("Front Panel Window:State")) -> (x = y?=w406:bool)
        n135 = Equal?(x=w414, y=T5."Run Time System" ("Application:Kind")) -> (x = y?=w412:bool)
        n136 = Or(x=w406, y=w412) -> (x .or. y?=w410:bool)
        n137 = Bundle By Name(cluster=w411, "Core.Current VI Reference"=w409, "Core.Close Panel on Exit?"=w410) -> (w415:T8)
        n138 = call <vilib>:"Add State(s) to Queue__JKI_lib_State_Machine.vi"("State(s) in (\"\")"=w417) -> ("States Out"=w416:string)  [unwired: 14 in]
      }
      frame "Exit" {
        n139 = call <vilib>:"Add State(s) to Queue__JKI_lib_State_Machine.vi"("State(s) in (\"\")"=w421) -> ("States Out"=w420:string)  [unwired: 14 in]
      }
      frame "---------- Data ----------" {
        n140 = call <vilib>:"Add State(s) to Queue__JKI_lib_State_Machine.vi"("State(s) in (\"\")"=w424) -> ("States Out"=w423:string)  [unwired: 14 in]
      }
      frame "Data: Initialize" {
        w425 = T7 {"Current VI Reference"=refnum, "Close Panel on Exit?"=FALSE}  # Core
        w426 = TRUE  # Your Boolean data
        n141 = Bundle("Core"=w425, "Your Boolean data"=w426) -> (w427:T8)  [unwired: 1 in]
        n142 = call <vilib>:"Add State(s) to Queue__JKI_lib_State_Machine.vi"("State(s) in (\"\")"=w429) -> ("States Out"=w428:string)  [unwired: 14 in]
      }
      frame "Data: Get Configuration", "Data: Get Internal Data" {
        n143 = call "Query Data as API String Arguments.vim"("Name"=w430, "Cluster Data"=w434) -> ("error"=w431:errorcluster, "API String"=w432:string, "Cluster Data (dup)"=w433:T8)  [unwired: 7 in]
      }
      frame "Data: Set Configuration" {
        n144 = call "Convert API String Arguments to Data.vim"("Reference Type"=w438, "API String"=w439) -> ("error out"=w436:errorcluster, "Data"=w437:T8)  [unwired: 6 in]
      }
      frame "Data: Update Indicators" {
      }
      frame "Data: Cleanup" {
        n145 = Unbundle By Name(w443) -> ("Core.Current VI Reference"=w445:refnum<vi>)
        n146 = Close Reference(reference=w445) -> (error out=w444:errorcluster)  [unwired: 1 in]
        n147 = call <vilib>:"Add State(s) to Queue__JKI_lib_State_Machine.vi"("State(s) in (\"\")"=w447) -> ("States Out"=w446:string)  [unwired: 14 in]
      }
      frame "---------- Macro ----------" {
        n148 = call <vilib>:"Add State(s) to Queue__JKI_lib_State_Machine.vi"("State(s) in (\"\")"=w450) -> ("States Out"=w449:string)  [unwired: 14 in]
      }
      frame "Macro: Initialize" {
        n149 = call <vilib>:"Add State(s) to Queue__JKI_lib_State_Machine.vi"("State(s) in Front (\"\")"="Data: Initialize\nInitialize Core Data\nData: Update Indicators", "State(s) in (\"\")"=w454) -> ("States Out"=w453:string)  [unwired: 13 in]
      }
      frame "Macro: Exit" {
        n150 = call <vilib>:"Add State(s) to Queue__JKI_lib_State_Machine.vi"("State(s) in Front (\"\")"="Data: Cleanup\nExit", "State(s) in (\"\")"=w458) -> ("States Out"=w457:string)  [unwired: 13 in]
      }
      frame "---------- API ----------" {
      }
      frame "API: API1" {
      }
      frame "API: API2" {
        # "unpack Hex String  to Variant\nif complex parameter is needed."
        n151 = call <userlib>:"CSM - Convert HexStr to Data.vi"("HEX String"=w465) -> ()  [unwired: 7 in, 2 out]
        n152 = disable-structure shown="Enabled" {
          disable-tunnel: [w468 "API2 Response"] -> w464
          frame Disabled {
            # "pack variant to hexstr \nif complex response is needed."
            # "complex Response"
            n153 = call <userlib>:"CSM - Convert Data to HexStr.vi"() -> ("HEX String (0-9,A-F)"=w468:string)  [unwired: 9 in]
          }
          frame Enabled {
          }
        }
      }
      frame "---------- Action ----------" {
        n154 = call <vilib>:"Add State(s) to Queue__JKI_lib_State_Machine.vi"("State(s) in (\"\")"=w472) -> ("States Out"=w471:string)  [unwired: 14 in]
      }
      frame "Action: Send Sync Message" {
        n155 = call <vilib>:"Add State(s) to Queue__JKI_lib_State_Machine.vi"("State(s) in (\"\")"=w475) -> ("States Out"=w474:string)  [unwired: 14 in]
      }
    }
  }
  n156 = call <vilib>:"Clear Errors.vi"("error in (no error)"=w13) -> ("error out"=w12:errorcluster)  [unwired: 5 in, 1 out]
  n157 = call <userlib>:"CSM - Send Message and Wait for Reply.vi"("Error In (No Error)"=w12, "Target Module"=w3, "State"="Macro: Exit") -> ()  [unwired: 6 in, 3 out]
